vi "Trim_Filename_DOS.vi"(1 "Input string":string, 2 "length":i32=7) -> (0 "output string":string)   [LabVIEW 2020]
panel:
  out "after substring":string
  out "before substring":string
  out "match substring":string
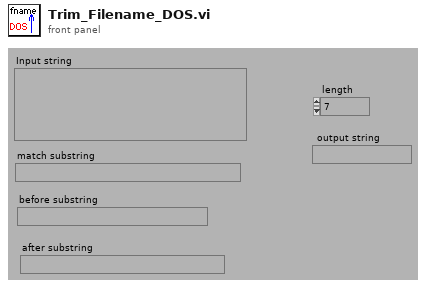
[diagram p1: front panel]
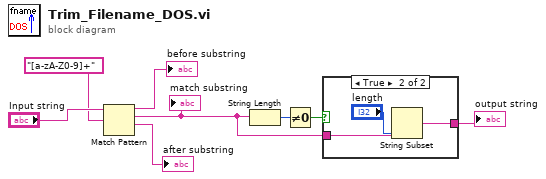
[diagram p0: block diagram]
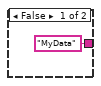
[diagram p2: hidden frame]
diagram:
  n1 = Match Pattern(string="Input string", regular expression="[a-zA-Z0-9]+") -> (before substring=→"before substring":string, match substring=w2:string, after substring=→"after substring":string)  [unwired: 1 in, 1 out]
  "match substring" <- w2
  n2 = String Length(string=w2) -> (length=w3:i32)
  n3 = Not Equal To 0?(x=w3) -> (x != 0?=w4:bool)
  n4 = case shown="True" w4 {
    tunnel: w2 -> [_ w12]
    tunnel: ["MyData" w11] -> w1
    frame False {
    }
    frame True {
      n5 = String Subset(string=w12, length (rest)="length") -> (substring=w11:string)  [unwired: 1 in]
    }
  }
  "output string" <- w1
